vi "SubVI_Circle Auto #.vi"(8 "error in":errorcluster, 10 "Parameter_Circle":T3={"ROI Descriptor"={"Global Rectangle"=[], "Contours"=[]}, "Edge Options"={"Edge Polarity"=0, "Kernel Size"=3, "Width"=3, "Minimum Edge Strength"=10.0, "Interpolation Type"=enum."Bilinear Fixed", "Data Processing Method"=enum."Average"}, "Scan Direction"=0, "Step Size"=5.0, "Auto"=FALSE, "Standard deviation"=0.0} {"Scan Direction" items=["Outside To Inside", "Inside To Outside"]; "Edge Options"."Edge Polarity" items=["All Edges", "Rising Edges", "Falling Edges"]; "Edge Options"."Minimum Edge Strength" format="%.2f"; "Edge Options"."Width" step=2; "Edge Options"."Kernel Size" step=2; "ROI Descriptor"."Contours"."Type" items=["No Selection", "Point", "Line", "Rectangle", "Oval", "Polygon", "Free", "Annulus", "Unused2", "Unused3", "Broken Line", "Free Hand Line", "Rotated Rectangle"]}, 11 "Image in":T5) -> (0 "error out":errorcluster, 2 "Result_Circle":T4 {"Center"."Y" format="%.2f"; "Center"."X" format="%.2f"}, 3 "Image Out":T5)   [LabVIEW 2013]
uses:
  <vilib>/vision/Image Controls.llb/IMAQ Image.ctl
  <vilib>/vision/Measure.llb/Edge Options.ctl
  <vilib>/vision/Measure.llb/Edge Polarity.ctl
  <vilib>/Analysis/NI_AALBase.lvlib
  <vilib>/vision/NI_Vision_Development_Module.lvlib
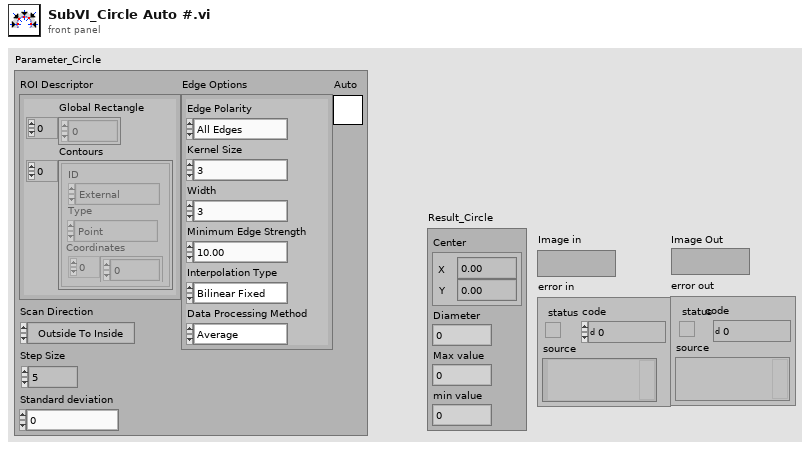
[diagram p1: front panel]
types:
  T1 = typedef "Edge Options.ctl" = cluster{"Edge Polarity":T2, "Kernel Size":u32, "Width":u32, "Minimum Edge Strength":sgl, "Interpolation Type":enum32{"Zero Order", "Bilinear", "Quadratic", "Cubic", "Bilinear Fixed"}, "Data Processing Method":enum32{"Average", "Median"}}
  T2 = typedef "Edge Polarity.ctl" = u32
  T3 = cluster{"ROI Descriptor":cluster{"Global Rectangle":i32[], "Contours":cluster{"ID":enum32{"External", "Internal"}, "Type":u32, "Coordinates":i32[]}[]}, "Edge Options":T1, "Scan Direction":u16, "Step Size":dbl, "Auto":bool, "Standard deviation":dbl}
  T4 = cluster{"Center":cluster{"X":sgl, "Y":sgl}, "Diameter":dbl, "Max value":sgl, "min value":sgl}
  T5 = typedef "IMAQ Image.ctl" = refnum<image>
  T6 = cluster{"Center":cluster{"X":sgl, "Y":sgl}, "Radius":dbl}
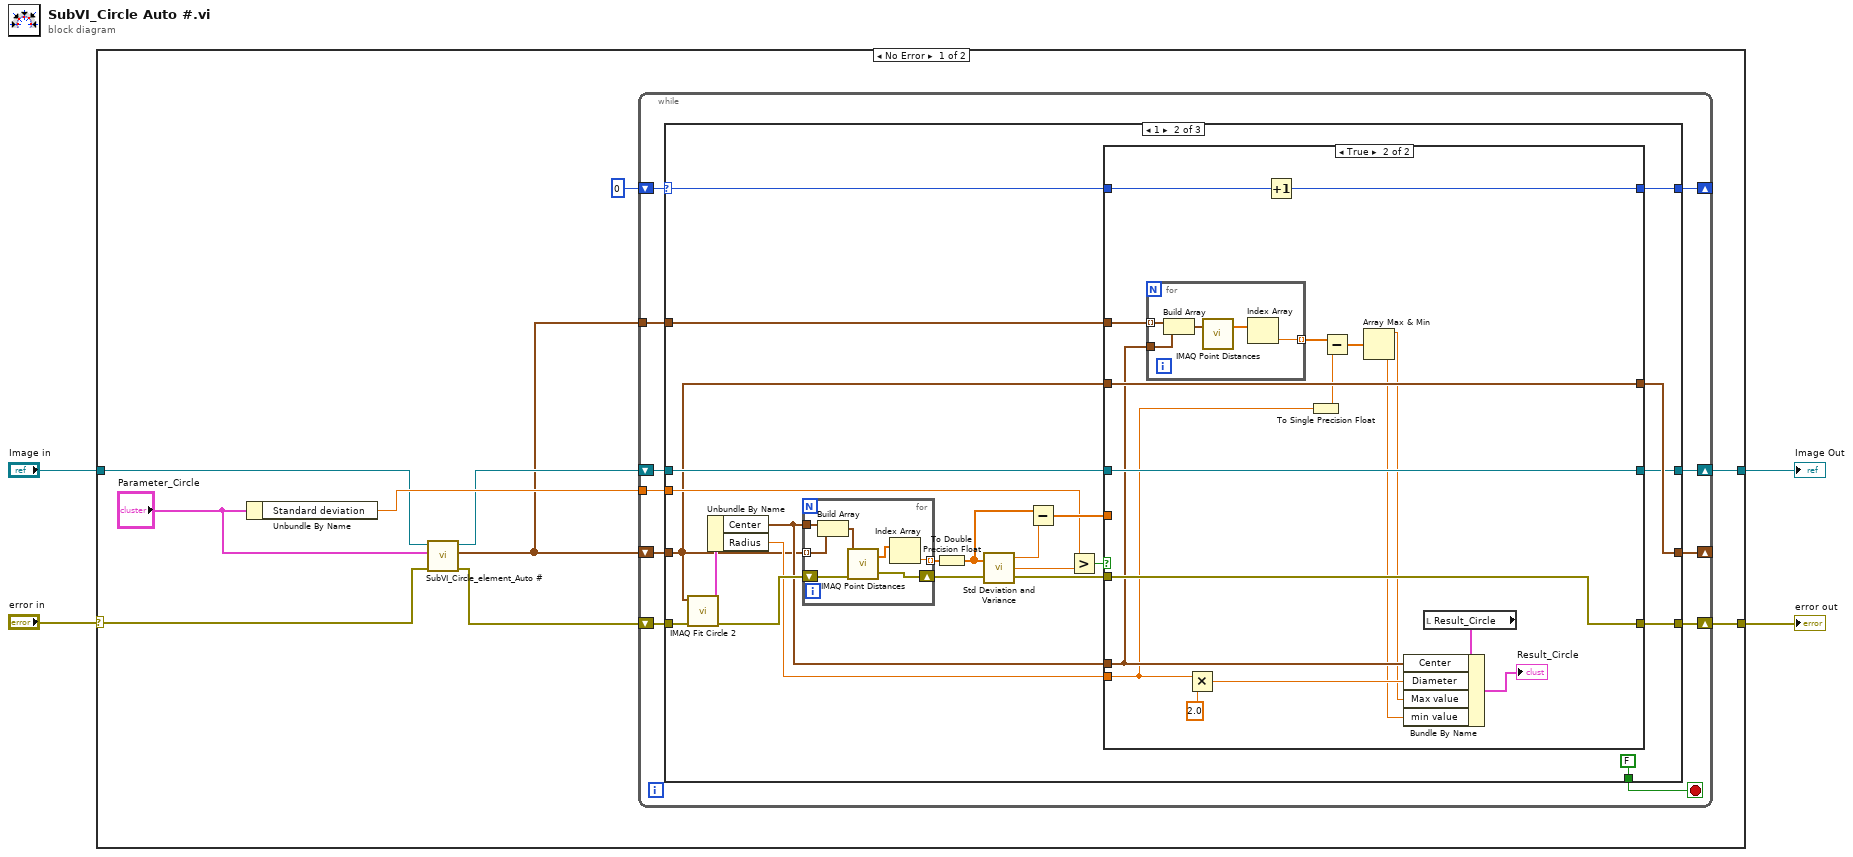
[diagram p0: block diagram]
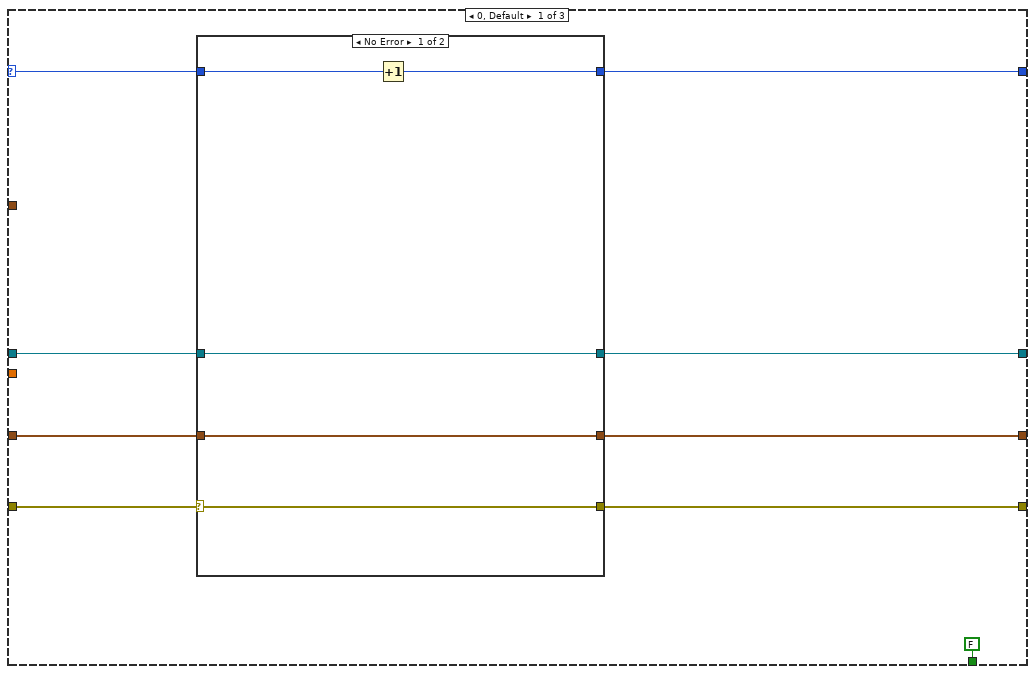
[diagram p2: hidden frame]
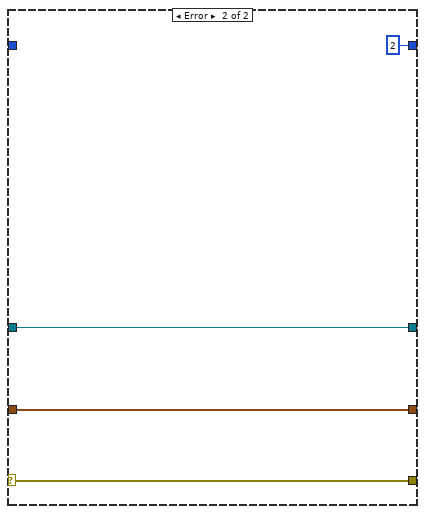
[diagram p3: hidden frame]
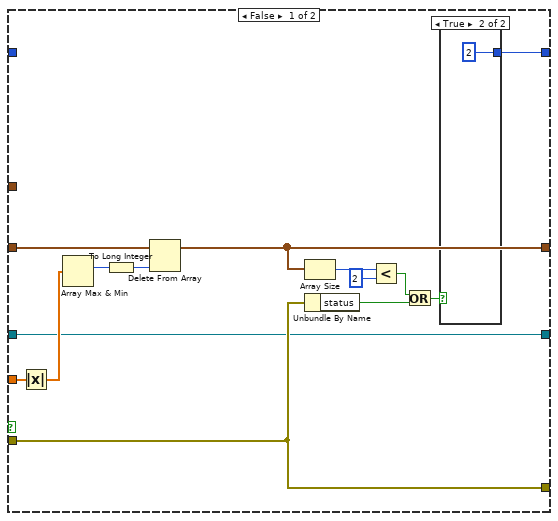
[diagram p4: hidden frame]
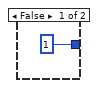
[diagram p5: hidden frame]
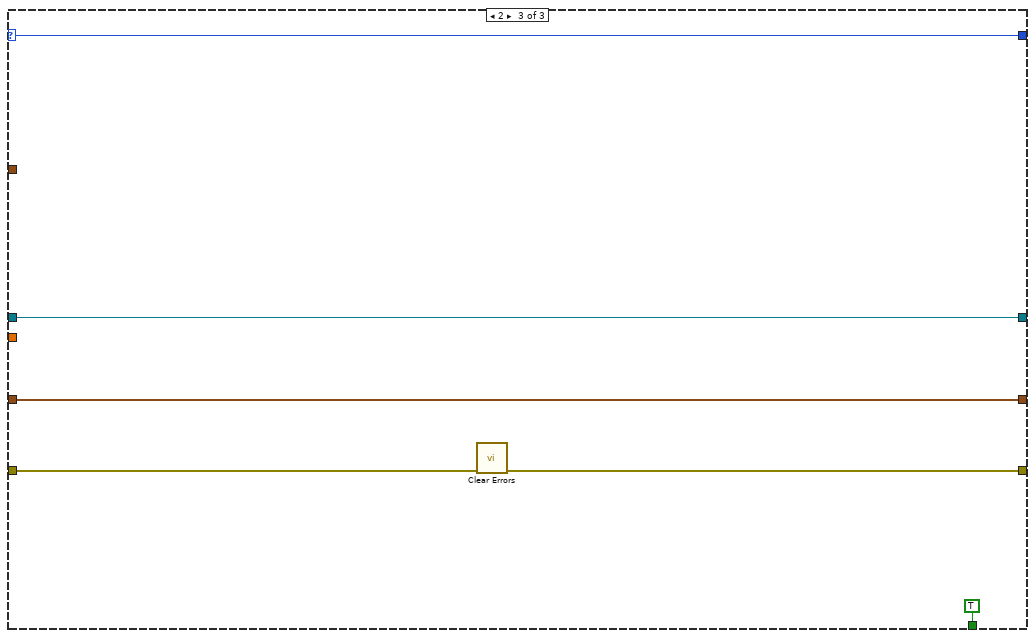
[diagram p6: hidden frame]
diagram:
  n1 = case shown="No Error" "error in" {
    selector: "error in" -> [w7 w118]
    tunnel: [w13 w118] -> w4
    tunnel: [w12 w117] -> w3
    tunnel: "Image in" -> [w9 w117]
    frame No Error {
      n2 = Unbundle By Name("Parameter_Circle") -> ("Standard deviation"=w11:dbl)
      n3 = call "SubVI_Circle_element_Auto #.vi"("Error In"=w7, "Parameter_Circle"="Parameter_Circle", "Image In"=w9) -> ("Error Out"=w8:errorcluster, "Location"=w5:cluster{"X":sgl, "Y":sgl}[], "Image Out"=w10:T5)  [unwired: 6 in]
      n4 = while {
        shift-right: [w23] -> _
        shift-left: 0 -> [w25]
        shift-right: [w22] -> w13
        shift-left: w8 -> [w24]
        shift-right: [w20] -> _
        shift-left: w5 -> [w21]
        shift-right: [w18] -> w12
        shift-left: w10 -> [w19]
        tunnel: w11 -> [w16]
        tunnel: w5 -> [w15]
        stop <- w17 stop-if-true
        n5 = case shown="1" w25 {
          selector: w25 -> [w30 w55 w111]
          tunnel: w24 -> [w28 w64 w116]
          tunnel: [w29 w56 w111] -> w23
          tunnel: [w32 w57 w115] -> w22
          tunnel: [w26 w61 w113] -> w20
          tunnel: w21 -> [w27 w45 w113]
          tunnel: w19 -> [w34 w60 w114]
          tunnel: [w33 w59 w114] -> w18
          tunnel: [FALSE FALSE TRUE] -> w17
          tunnel: w16 -> [_ w46 _]
          tunnel: w15 -> [_ w44 _]
          frame 0, Default {
            n6 = case shown="No Error" w28 {
              selector: w28 -> [w35 w41]
              tunnel: w34 -> [w36 w42]
              tunnel: [w36 w42] -> w33
              tunnel: [w35 w41] -> w32
              tunnel: w30 -> [w39 _]
              tunnel: [w38 2] -> w29
              tunnel: w27 -> [w37 w40]
              tunnel: [w37 w40] -> w26
              frame No Error {
                n7 = Increment(x=w39) -> (x+1=w38:i32)
              }
              frame Error {
              }
            }
          }
          frame 1 {
            n8 = call "IMAQ Fit Circle 2"("error in (no error)"=w64, "Radial Points"=w45) -> ("error out"=w63:errorcluster, "Circle"=w52:T6)  [unwired: 4 in, 4 out]
            n9 = Unbundle By Name(w52) -> ("Center"=w48:cluster{"X":sgl, "Y":sgl}, "Radius"=w47:dbl)
            n10 = for {
              tunnel: [w104] -> w51 mode=indexing
              shift-right: [w109] -> w58
              shift-left: w63 -> [w110]
              tunnel: w48 -> [w108]
              tunnel: w45 -> [w107] mode=indexing
              n11 = Build Array(w108, w107) -> (w106:cluster{"X":sgl, "Y":sgl}[])
              n12 = call "IMAQ Point Distances"("Points"=w106, "error in (no error)"=w110) -> ("Distances"=w105:sgl[], "error out"=w109:errorcluster)  [unwired: 3 in]
              n13 = Index Array(array=w105) -> (element=w104:sgl)  [unwired: 1 in]
            }
            n14 = To Double Precision Float(number=w51) -> (double precision float=w50:dbl[])
            n15 = call <vilib>:"Std Deviation and Variance.vi"("X"=w50) -> ("mean"=w49:dbl, "standard deviation"=w65:dbl)  [unwired: 1 in, 1 out]
            n16 = Subtract(x=w50, y=w49) -> (x-y=w54:dbl[])
            n17 = Greater?(x=w46, y=w65) -> (0:w62:bool)
            n18 = case shown="True" w62 {
              tunnel: w45 -> [w79 w96]
              tunnel: [w74 w96] -> w61
              tunnel: w60 -> [w66 w92]
              tunnel: [w66 w92] -> w59
              tunnel: w58 -> [w67 w91]
              tunnel: [w67 w91] -> w57
              tunnel: [w76 w97] -> w56
              tunnel: w55 -> [_ w98]
              tunnel: w54 -> [w68 _]
              tunnel: w48 -> [_ w88]
              tunnel: w47 -> [_ w86]
              tunnel: w44 -> [_ w89]
              frame False {
                n19 = Absolute Value(x=w68) -> (abs(x)=w69:dbl[])
                n20 = Array Max & Min(array=w69) -> (max index (indices)=w78:i32)  [unwired: 3 out]
                n21 = To Long Integer(number=w78) -> (32bit integer=w77:i32)
                n22 = Delete From Array(array=w79, index=w77) -> (array with subset deleted=w74:cluster{"X":sgl, "Y":sgl}[])  [unwired: 1 in, 1 out]
                n23 = Array Size(array=w74) -> (size(s)=w73:i32)
                n24 = Unbundle By Name(w67) -> ("status"=w75:bool)
                n25 = Less?(x=w73, y=2) -> (x < y?=w71:bool)
                n26 = Or(x=w71, y=w75) -> (x .or. y?=w70:bool)
                n27 = case shown="True" w70 {
                  tunnel: [1 2] -> w76
                  frame False {
                  }
                  frame True {
                  }
                }
              }
              frame True {
                n28 = for {
                  tunnel: w89 -> [w103] mode=indexing
                  tunnel: w88 -> [w102]
                  tunnel: [w99] -> w87 mode=indexing
                  n29 = Build Array(w103, w102) -> (w101:cluster{"X":sgl, "Y":sgl}[])
                  n30 = call "IMAQ Point Distances"("Points"=w101) -> ("Distances"=w100:sgl[])  [unwired: 4 in, 1 out]
                  n31 = Index Array(array=w100) -> (element=w99:sgl)  [unwired: 1 in]
                }
                n32 = Multiply(x=w86, y=2.0) -> (x*y=w90:dbl)
                n33 = Increment(x=w98) -> (x+1=w97:i32)
                n34 = To Single Precision Float(number=w86) -> (single precision float=w85:sgl)
                n35 = Subtract(x=w87, y=w85) -> (x-y=w84:sgl[])
                n36 = Array Max & Min(array=w84) -> (max value=w83:sgl, min value=w82:sgl)  [unwired: 2 out]
                n37 = local read "Result_Circle"() -> (w94:T4)
                n38 = Bundle By Name(cluster=w94, "Center"=w88, "Diameter"=w90, "Max value"=w83, "min value"=w82) -> (→"Result_Circle":T4)
              }
            }
          }
          frame 2 {
            n39 = call <vilib>:"Clear Errors.vi"("error in (no error)"=w116) -> ("error out"=w115:errorcluster)  [unwired: 6 in]
          }
        }
      }
    }
    frame Error {
    }
  }
  "error out" <- w4
  "Image Out" <- w3
